vi "Ellipse fit.vi"() -> ()   [LabVIEW 2023]
doc: "This demonstrates how to use nonlinear curve fitting to fit an ellipse. \nThis problem is modelled as a 2D curve fit (2 domains, 1 range), \nwhere the X and Y data are the noisy points, and Z is 1."
uses:
  <vilib>/gmath/NumericalOptimization/Nonlinear Curve Fit LM.vi
  <vilib>/gmath/NI_Gmath.lvlib
  <vilib>/Analysis/NI_AALBase.lvlib
panel:
  out "XY Graph":cluster{"X":dbl[], "Y":dbl[]}[](graph)
  out "fit y0":dbl
  out "fit x0":dbl
  out "fit b":dbl
  out "fit a":dbl
  in  "b":dbl=0.3
  out "#function calls":i32
  out "residue":dbl
  in  "noise sigma":dbl=0.021 format="%#.6g"
  in  "a":dbl=0.6
  in  "y0":dbl=0.2
  in  "x0":dbl=0.1
  # "Overview: Demonstrates how to use the Nonlinear Curve Fit VI to fit an ellipse. \nRequirements: LabVIEW Full Development System\nInstructions:\n1. Run the VI.\n2. Change some of the ellipse parameters and run the VI again."
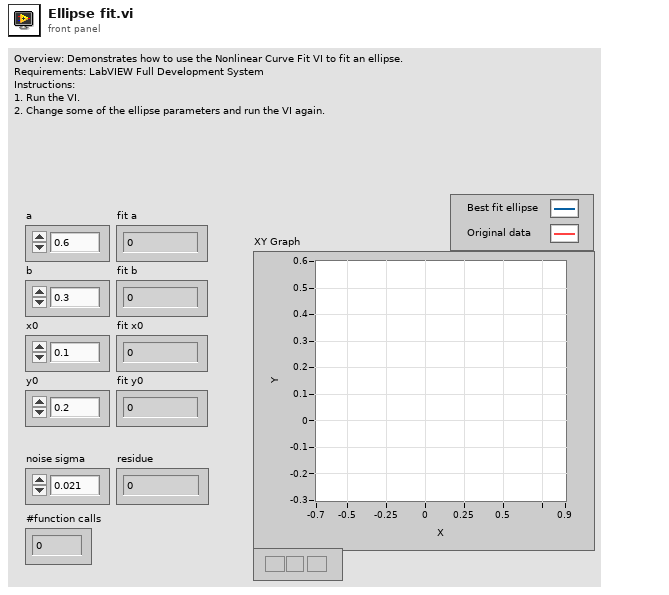
[diagram p1: front panel]
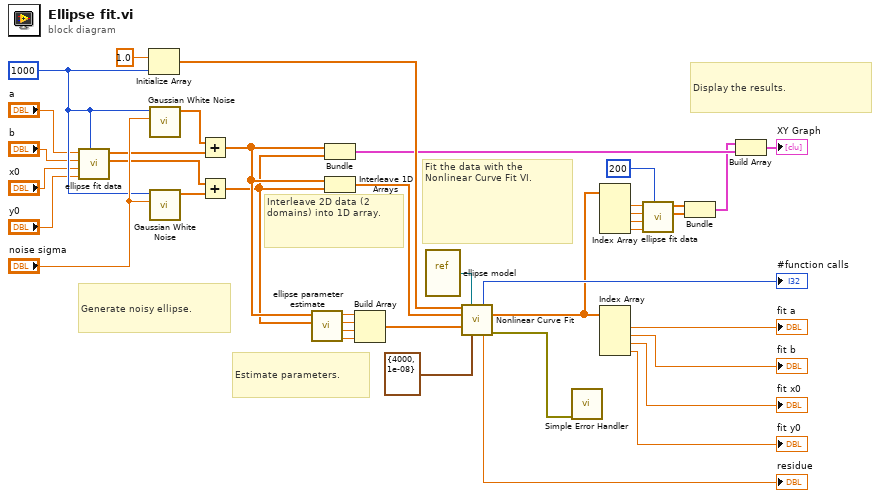
[diagram p0: block diagram]
diagram:
  w39 = 1000 ("samples")
  # "Estimate parameters."
  # "Display the results."
  # "Fit the data with the Nonlinear Curve Fit VI."
  # "Interleave 2D data (2 domains) into 1D array."
  # "Generate noisy ellipse."
  n1 = call "ellipse fit data.vi"("samples"=w39, "y0"="y0", "x0"="x0", "b"="b", "a"="a") -> ("Y"=w26:dbl[], "X"=w25:dbl[])  [unwired: 5 in]
  n2 = Initialize Array(1.0, w39) -> (w22:dbl[])
  n3 = call <vilib>:"Gaussian White Noise.vi"("standard deviation"="noise sigma", "samples"=w39) -> ("Gaussian noise pattern"=w36:dbl[])  [unwired: 8 in, 1 out]
  n4 = call <vilib>:"Gaussian White Noise.vi"("standard deviation"="noise sigma", "samples"=w39) -> ("Gaussian noise pattern"=w35:dbl[])  [unwired: 8 in, 1 out]
  n5 = Add(x=w36, y=w25) -> (x+y=w10:dbl[])
  n6 = Add(x=w26, y=w35) -> (x+y=w9:dbl[])
  n7 = call "ellipse parameter estimate.vi"("Y"=w9, "X"=w10) -> ("y0"=w14:dbl, "x0"=w15:dbl, "b"=w16:dbl, "a"=w17:dbl)  [unwired: 6 in]
  n8 = Bundle(w10, w9) -> (w3:cluster{dbl[], dbl[]})  [unwired: 1 in]
  n9 = Interleave 1D Arrays(w10, w9) -> (w31:dbl[])
  n10 = Build Array(w17, w16, w15, w14) -> (w29:dbl[])
  n11 = vi-ref "ellipse model.vi"() -> (w27:refnum<vi>)
  n12 = call-poly <vilib>:"Nonlinear Curve Fit.vi"("Y"=w22, "f(x,a)"=w27, "X"=w31, "initial parameters"=w29, "termination"=cluster{"max iteration":i32, "tolerance":dbl} {"max iteration"=4000, "tolerance"=1e-08}) -> ("number of function calls"=→"#function calls":i32, "best fit parameters"=w8:dbl[], "residue"=→"residue":dbl, "error out"=w1:errorcluster)  [unwired: 5 in, 2 out]
  n13 = call <vilib>:"Simple Error Handler.vi"("error in (no error)"=w1) -> ()  [unwired: 4 in, 5 out]
  n14 = Index Array(array=w8) -> (element #1=w24:dbl, element #2=w13:dbl, element #3=w12:dbl, element #4=w11:dbl)  [unwired: 4 in]
  n15 = Index Array(array=w8) -> (element #1=→"fit a":dbl, element #2=→"fit b":dbl, element #3=→"fit x0":dbl, element #4=→"fit y0":dbl)  [unwired: 4 in]
  n16 = call "ellipse fit data.vi"("samples"=200, "y0"=w11, "x0"=w12, "b"=w13, "a"=w24) -> ("Y"=w20:dbl[], "X"=w21:dbl[])  [unwired: 5 in]
  n17 = Bundle("X"=w21, "Y"=w20) -> (w2:cluster{"X":dbl[], "Y":dbl[]})  [unwired: 1 in]
  n18 = Build Array(w2, w3) -> (→"XY Graph":cluster{"X":dbl[], "Y":dbl[]}[])
